vi "LoadVisionPanel.vi"(8 "error in (no error)":errorcluster, 11 "MPC_VirbVision in":refnum<class "MPC_VirbVision.lvclass">) -> (0 "error out":errorcluster, 2 "This VI":refnum<vi>, 3 "MPC_VirbVision out":refnum<class "MPC_VirbVision.lvclass">)   [LabVIEW 2019, in "MPC_VirbVision.lvclass"]
uses:
  MPC_VirbVision.lvclass
  <vilib>/Utility/miscctls.llb/LVPointTypeDef.ctl
  Panel RefGlb.vi
panel:
  in  "Tab Control":enum32{"視覺", "震動盤", "IO", "視覺手臂校正"}(tab)
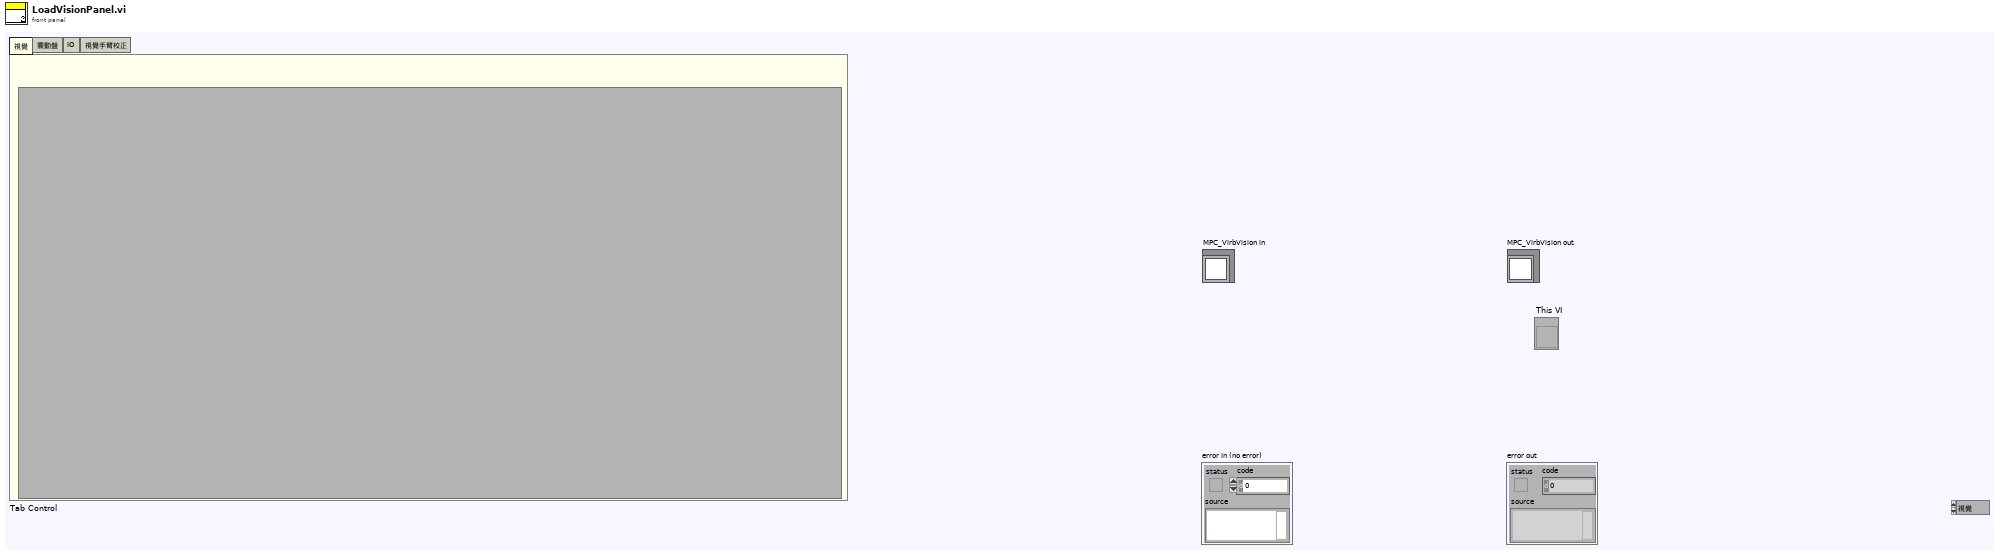
[diagram p1: front panel]
types:
  T1 = typedef "LVPointTypeDef.ctl" = cluster{"Horizontal":i16, "Vertical":i16}
  T2 = typedef "LVPositionTypeDef.ctl" = cluster{"Left":i32, "Top":i32}
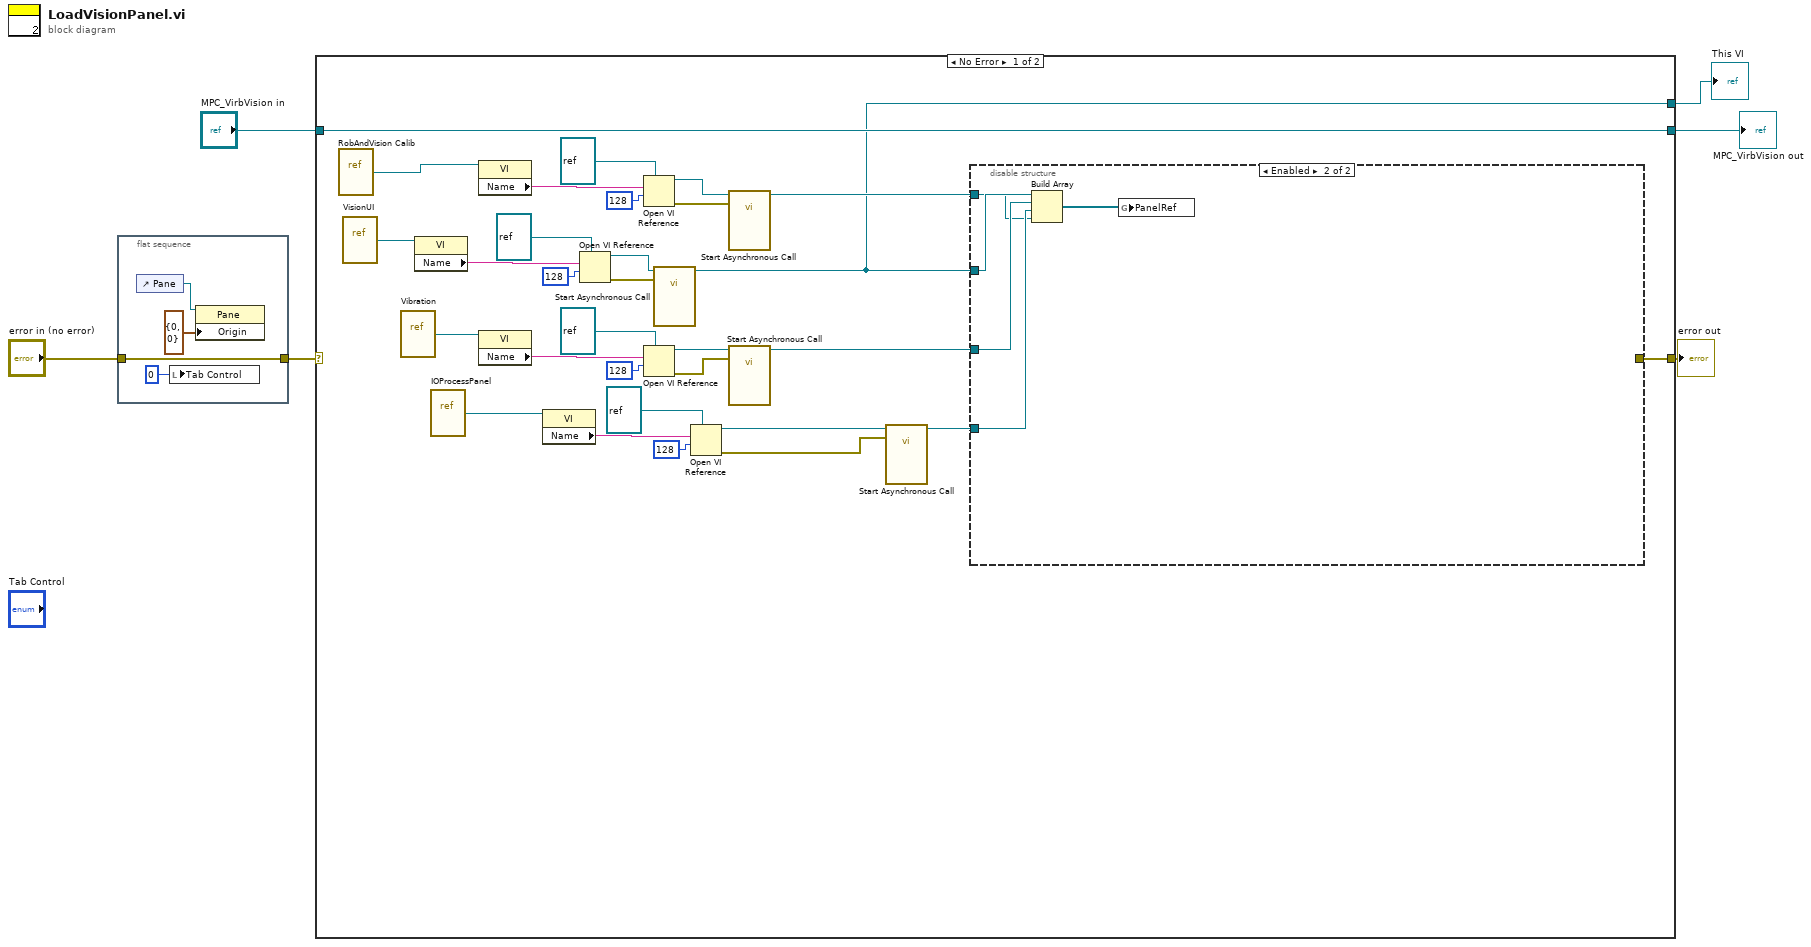
[diagram p0: block diagram]
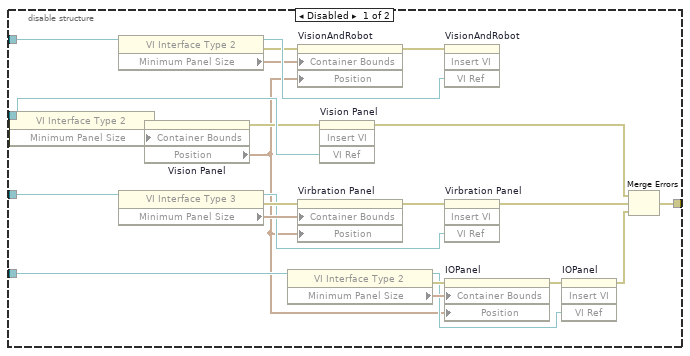
[diagram p2: hidden frame]
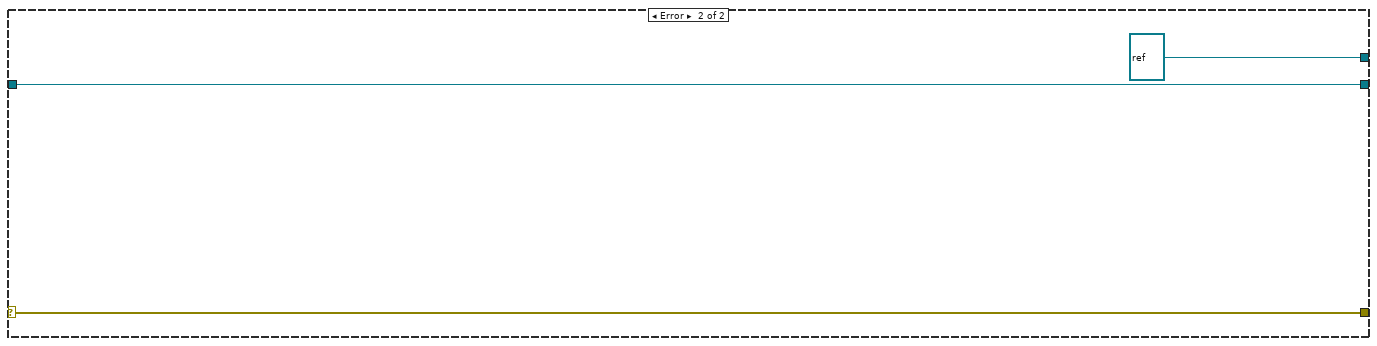
[diagram p3: hidden frame]
diagram:
  n1 = flat-sequence {
    tunnel: [w10] -> w1
    tunnel: "error in (no error)" -> [w10]
    frame #0 {
      n2 = control-ref of="Pane"() -> (w8:refnum<vi>)
      n3 = local write "Tab Control"(0) -> ()
      n4 = property class="Pane"(reference=w8, "Origin"=T1 {"Horizontal"=0, "Vertical"=0}) -> ()  [unwired: 1 in, 2 out]
    }
  }
  n5 = case shown="No Error" w1 {
    selector: w1 -> [_ w73]
    tunnel: [w11 refnum<vi> refnum ("type specifier VI Refnum (for type only)")] -> w6
    tunnel: [w19 w73] -> w5
    tunnel: [w34 w72] -> w4
    tunnel: "MPC_VirbVision in" -> [w34 w72]
    frame No Error {
      n6 = vi-ref "RobAndVision Calib.vi"() -> (w12:refnum<vi>)
      n7 = vi-ref "VisionUI.vi"() -> (w40:refnum<vi>)
      n8 = vi-ref "Vibration.vi"() -> (w27:refnum<vi>)
      n9 = property class="VI"(reference=w40) -> ("Name"=w39:string)  [unwired: 1 in, 2 out]
      n10 = vi-ref "IOProcessPanel.vi"() -> (w26:refnum<vi>)
      n11 = property class="VI"(reference=w12) -> ("Name"=w13:string)  [unwired: 1 in, 2 out]
      n12 = property class="VI"(reference=w27) -> ("Name"=w28:string)  [unwired: 1 in, 2 out]
      n13 = property class="VI"(reference=w26) -> ("Name"=w25:string)  [unwired: 1 in, 2 out]
      n14 = Open VI Reference(type specifier VI Refnum (for type only)=refnum<vi> refnum, vi path=w39, options=128) -> (vi reference=w37:refnum<vi>, error out=w36:errorcluster)  [unwired: 3 in]
      n15 = Open VI Reference(type specifier VI Refnum (for type only)=refnum<vi> refnum, vi path=w13, options=128) -> (vi reference=w15:refnum<vi>, error out=w16:errorcluster)  [unwired: 3 in]
      n16 = Open VI Reference(type specifier VI Refnum (for type only)=refnum<vi> refnum, vi path=w28, options=128) -> (vi reference=w30:refnum<vi>, error out=w31:errorcluster)  [unwired: 3 in]
      n17 = call-by-ref "Start Asynchronous Call"(reference=w37, error in=w36) -> (reference out=w11:refnum<vi>)  [unwired: 12 in, 1 out]
      n18 = Open VI Reference(type specifier VI Refnum (for type only)=refnum<vi> refnum, vi path=w25, options=128) -> (vi reference=w23:refnum<vi>, error out=w22:errorcluster)  [unwired: 3 in]
      n19 = call-by-ref "Start Asynchronous Call"(reference=w15, error in=w16) -> (reference out=w18:refnum<vi>)  [unwired: 12 in, 1 out]
      n20 = call-by-ref "Start Asynchronous Call"(reference=w30, error in=w31) -> (reference out=w33:refnum<vi>)  [unwired: 11 in, 2 out]
      n21 = call-by-ref "Start Asynchronous Call"(reference=w23, error in=w22) -> (reference out=w20:refnum<vi>)  [unwired: 12 in, 1 out]
      n22 = disable-structure shown="Enabled" {
        disable-tunnel: w11 -> [w65 w69]
        disable-tunnel: w33 -> [w58 w68]
        disable-tunnel: w20 -> [w57 w67]
        disable-tunnel: [w49 _] -> w19
        disable-tunnel: w18 -> [w42 w66]
        frame Disabled {
          n23 = property class="VI Interface Type 2"(reference=w65) -> (reference out=w62:refnum<vi>, error out=w63:errorcluster, "Minimum Panel Size"=w64:T1)  [unwired: 1 in]
          n24 = property class="VI Interface Type 2"(reference=w42) -> (reference out=w45:refnum<vi>, error out=w44:errorcluster, "Minimum Panel Size"=w43:T1)  [unwired: 1 in]
          n25 = property class="VI Interface Type 3"(reference=w58) -> (reference out=w54:refnum<vi>, error out=w60:errorcluster, "Minimum Panel Size"=w59:T1)  [unwired: 1 in]
          n26 = property on="Vision Panel" class="SubPnl"(error in=w63, "Container Bounds"=w64) -> (error out=w61:errorcluster, "Position"=w41:T2)  [unwired: 1 in, 1 out]
          n27 = property class="VI Interface Type 2"(reference=w57) -> (reference out=w53:refnum<vi>, error out=w55:errorcluster, "Minimum Panel Size"=w56:T1)  [unwired: 1 in]
          n28 = property on="VisionAndRobot" class="SubPnl"(error in=w44, "Container Bounds"=w43, "Position"=w41) -> (error out=w46:errorcluster)  [unwired: 1 in, 1 out]
          n29 = property on="Virbration Panel" class="SubPnl"(error in=w60, "Container Bounds"=w59, "Position"=w41) -> (error out=w47:errorcluster)  [unwired: 1 in, 1 out]
          n30 = invoke on="Vision Panel" class="SubPnl" method="Insert VI"(error in=w61, "VI Ref"=w62) -> (error out=w52:errorcluster)  [unwired: 2 in, 3 out]
          n31 = invoke on="VisionAndRobot" class="SubPnl" method="Insert VI"(error in=w46, "VI Ref"=w45) -> ()  [unwired: 2 in, 4 out]
          n32 = invoke on="Virbration Panel" class="SubPnl" method="Insert VI"(error in=w47, "VI Ref"=w54) -> (error out=w51:errorcluster)  [unwired: 2 in, 3 out]
          n33 = property on="IOPanel" class="SubPnl"(error in=w55, "Container Bounds"=w56, "Position"=w41) -> (error out=w48:errorcluster)  [unwired: 1 in, 1 out]
          n34 = invoke on="IOPanel" class="SubPnl" method="Insert VI"(error in=w48, "VI Ref"=w53) -> (error out=w50:errorcluster)  [unwired: 2 in, 3 out]
          n35 = Merge Errors(w52, w51, w50) -> (w49:errorcluster)
        }
        frame Enabled {
          n36 = Build Array(w69, w68, w67, w66) -> (w70:refnum<vi>[])
          n37 = global write "Panel RefGlb.vi" "PanelRef"(w70) -> ()
        }
      }
    }
    frame Error {
    }
  }
  "error out" <- w5
  "MPC_VirbVision out" <- w4
  "This VI" <- w6
